vi "Set magnet (oscillate).vi"(8 "错误输入（无错误）":errorcluster, 9 "Rate(Oe/s)":dbl, 10 "semaphore":T1, 11 "VISA引用句柄输入":refnum<visa-resource-name>) -> (0 "错误输出":errorcluster, 3 "VISA引用句柄输出":refnum<visa-resource-name>)   [LabVIEW 2019, in "9T cmag.lvlib"]
uses:
  9T cmag.lvlib
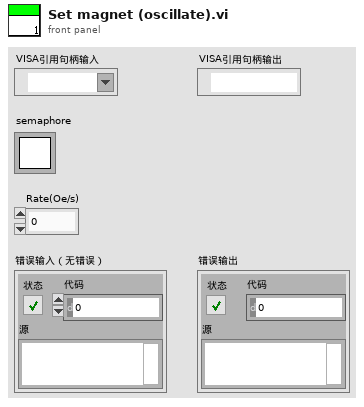
[diagram p1: front panel]
types:
  T1 = typedef "Semaphore RefNum" = refnum<k1>
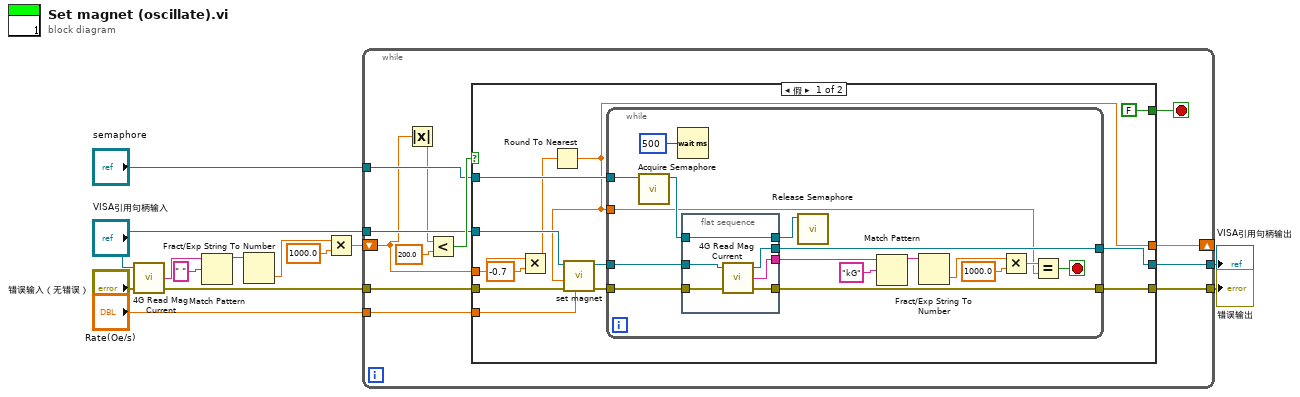
[diagram p0: block diagram]
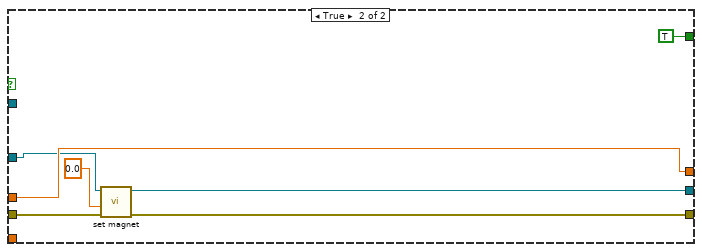
[diagram p2: hidden frame]
diagram:
  n1 = call "4G Read Mag Current.vi"("error in (no error)"="错误输入（无错误）", "VISA session"="VISA引用句柄输入") -> ("error out"=w5:errorcluster, "response out"=w1:string)  [unwired: 1 in, 1 out]
  n2 = Match Pattern(string=w1, regular expression=" " ("正则表达式")) -> (before substring=w4:string)  [unwired: 1 in, 3 out]
  n3 = Fract/Exp String To Number(string=w4) -> (number=w9:dbl)  [unwired: 3 in, 1 out]
  n4 = Multiply(x=w9, y=1000.0) -> (x*y=w10:dbl)
  n5 = while {
    shift-right: [w21] -> _
    shift-left: w10 -> [w16]
    tunnel: "VISA引用句柄输入" -> [w22]
    tunnel: w5 -> [w20]
    tunnel: [w19] -> w8
    tunnel: [w18] -> w7
    tunnel: "semaphore" -> [w17]
    tunnel: "Rate(Oe/s)" -> [w14]
    stop <- w23 stop-if-true
    n6 = Absolute Value(x=w16) -> (abs(x)=w15:dbl)
    n7 = Less?(x=w15, y=200.0) -> (x < y?=w24:bool)
    n8 = case shown="假" w24 {
      tunnel: [FALSE TRUE] -> w23
      tunnel: w22 -> [w37 w65]
      tunnel: w16 -> [w35 w66]
      tunnel: [w27 w66] -> w21
      tunnel: w20 -> [w33 w63]
      tunnel: [w31 w62] -> w19
      tunnel: [w30 w61] -> w18
      tunnel: w17 -> [w29 _]
      tunnel: w14 -> [w26 _]
      frame False {
        n9 = Multiply(x=w35, y=-0.7) -> (x*y=w28:dbl)
        n10 = Round To Nearest(number=w28) -> (nearest integer value=w27:dbl)
        n11 = call "set magnet.vi"("Rate(Oe/s)"=w26, "error in (no error)"=w33, "Magnet field(Oe)"=w27, "VISA Resource Name"=w37) -> ("error out"=w32:errorcluster, "dup VISA session"=w34:refnum<visa-resource-name>)  [unwired: 5 in, 1 out]
        n12 = while {
          tunnel: w34 -> [w53]
          tunnel: w32 -> [w52]
          tunnel: [w50] -> w31
          tunnel: [w51] -> w30
          tunnel: w29 -> [w48]
          tunnel: w27 -> [w39]
          stop <- w40 stop-if-true
          n13 = call <vilib>:"Acquire Semaphore.vi"("semaphore"=w48) -> ("semaphore out"=w49:T1)  [unwired: 4 in, 2 out]
          n14 = Wait (ms)(milliseconds to wait=u32 500) -> ()  [unwired: 1 out]
          n15 = flat-sequence {
            tunnel: w53 -> [w60]
            tunnel: w52 -> [w59]
            tunnel: [w58] -> w51
            tunnel: [w57] -> w50
            tunnel: w49 -> [w56]
            tunnel: [w56] -> w47
            tunnel: [w55] -> w46
            frame #0 {
              n16 = call "4G Read Mag Current.vi"("error in (no error)"=w59, "VISA session"=w60) -> ("error out"=w57:errorcluster, "response out"=w55:string, "dup VISA session"=w58:refnum<visa-resource-name>)  [unwired: 1 in]
            }
          }
          n17 = call <vilib>:"Release Semaphore.vi"("semaphore"=w47) -> ()  [unwired: 5 in, 2 out]
          n18 = Match Pattern(string=w46, regular expression="kG") -> (before substring=w44:string)  [unwired: 1 in, 3 out]
          n19 = Fract/Exp String To Number(string=w44) -> (number=w43:dbl)  [unwired: 3 in, 1 out]
          n20 = Multiply(x=w43, y=1000.0) -> (x*y=w41:dbl)
          n21 = Equal?(x=w41, y=w39) -> (x = y?=w40:bool)
        }
      }
      frame True {
        n22 = call "set magnet.vi"("error in (no error)"=w63, "Magnet field(Oe)"=0.0, "VISA Resource Name"=w65) -> ("error out"=w62:errorcluster, "dup VISA session"=w61:refnum<visa-resource-name>)  [unwired: 6 in, 1 out]
      }
    }
  }
  "错误输出" <- w8
  "VISA引用句柄输出" <- w7
